vi "Remote Client.vi"(6 "Wait for Response? [T]":bool=TRUE, 8 "error in (no error)":errorcluster, 9 "Data":variant, 10 "Command":string, 11 "Instrument in":refnum<class "Instrument.lvclass">) -> (0 "error out":errorcluster, 1 "Data out":variant, 2 "Command out":string, 3 "Instrument out":refnum<class "Instrument.lvclass">)   [LabVIEW 2016, in "Instrument.lvclass"]
uses:
  Instrument.lvclass
  Instrument.lvclass/Instrument.ctl
  RemoteControl/RemoteControl.lvclass
  RemoteControl.STM/RemoteControl.STM.lvclass
  C:/user/patrick/hg/levylab_inst/lvsrc/SMOs/RemoteControl/RemoteControl.lvclass
  <userlib>/_OpenG.lib/numeric/numeric.llb/Random Number Within Range - I32__ogtk.vi
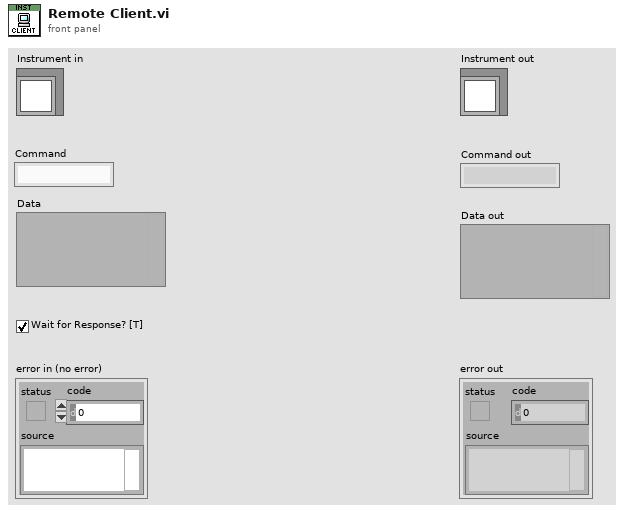
[diagram p1: front panel]
types:
  T1 = typedef "Instrument.lvclass/PublicEvents--Cluster.ctl" = cluster{"MessageFromProcess":refnum<user-event>}
  T2 = typedef "Instrument.lvclass/SMO RC Type--enum.ctl" = enum16{"RC", "STM", "ZMQ"}
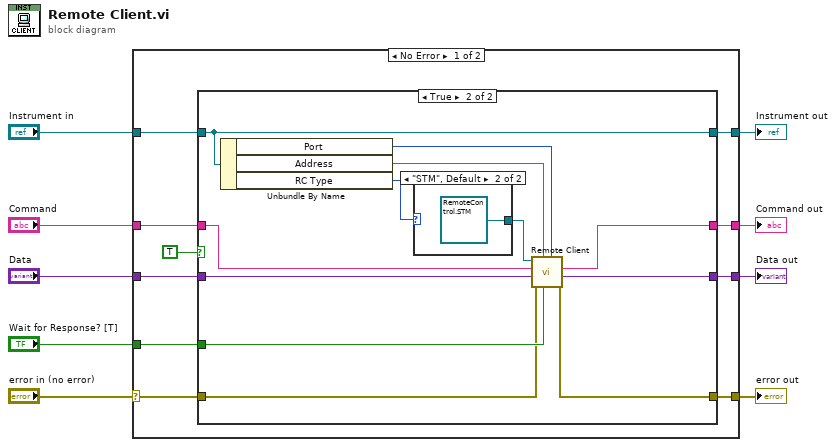
[diagram p0: block diagram]
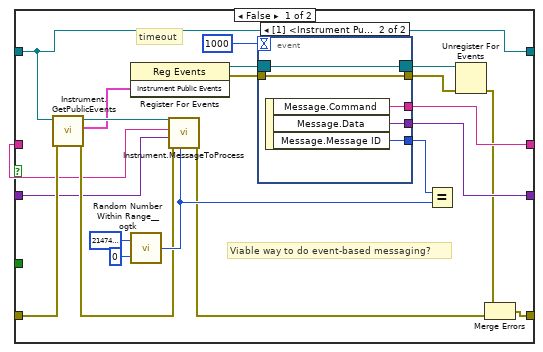
[diagram p2: hidden frame]
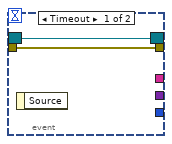
[diagram p3: hidden frame]
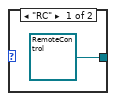
[diagram p4: hidden frame]
diagram:
  n1 = case shown="No Error" "error in (no error)" {
    selector: "error in (no error)" -> [w19 w64]
    tunnel: [w18 w64] -> w8
    tunnel: [w10 w63] -> w6
    tunnel: "Instrument in" -> [w11 w63]
    tunnel: [w17 _] -> w5
    tunnel: [w13 w62] -> w4
    tunnel: "Command" -> [w14 w62]
    tunnel: "Data" -> [w16 _]
    tunnel: "Wait for Response? [T]" -> [w15 _]
    frame No Error {
      n2 = case shown="True" TRUE {
        tunnel: w19 -> [w29 w52]
        tunnel: [w22 w59] -> w18
        tunnel: [w35 w58] -> w17
        tunnel: w16 -> [w27 w57]
        tunnel: w15 -> [_ w56]
        tunnel: w11 -> [w20 w48]
        tunnel: w14 -> [w26 w53]
        tunnel: [w25 w54] -> w13
        tunnel: [w20 w48] -> w10
        frame False {
          # "Viable way to do event-based messaging?"
          # "timeout"
          n3 = call "Instrument.GetPublicEvents.vi"("error in (no error)"=w29, "Instrument"=w20) -> ("error out"=w28:errorcluster, "Instrument Public Events"=w37:T1, "Instrument out"=w38:refnum<class "Instrument.lvclass">)  [unwired: 7 in]
          n4 = register-events(w37) -> (reference out=w36:refnum<event-registration>, error out=w32:errorcluster)  [unwired: 2 in]
          n5 = call-poly <userlib>:"Random Number Within Range__ogtk.vi"("High"=2147483647, "Low"=0) -> ("Random Number"=w31:i32)  [unwired: 3 in]
          n6 = call "Instrument.MessageToProcess.vi"("Message ID"=w31, "error in (no error)"=w28, "Message.Data"=w27, "Message.Command"=w26, "Instrument"=w38) -> ("error out"=w21:errorcluster)  [unwired: 5 in, 1 out]
          n7 = event shown="[1] <Instrument Public Events.MessageFromProcess>: User Event" {
            selector: w36 -> [w41 w43]
            dyn-events: [w41 w43] -> w24
            timeout: 1000 -> [_ _]
            tunnel: [_ w47] -> w25
            tunnel: [_ w46] -> w35
            tunnel: [w42 w45] -> w33
            tunnel: w32 -> [w42 w45]
            tunnel: [_ w44] -> w30
            event Timeout {
              n8 = event-data() -> ()  [unwired: 1 in, 1 out]
            }
            event User Event {
              n9 = event-data() -> ("Message.Command"=w47:string, "Message.Data"=w46:variant, "Message.Message ID"=w44:i32)  [unwired: 1 in]
            }
          }
          n10 = Equal?(x=w30, y=w31) -> ()  [unwired: 1 out]
          n11 = Unregister For Events(event registration refnum=w24, error in=w33) -> (error out=w23:errorcluster)
          n12 = Merge Errors(w23, w21) -> (w22:errorcluster)
        }
        frame True {
          n13 = Unbundle By Name(w48) -> ("Port"=w51:u16, "Address"=w55:string, "RC Type"=w49:T2)
          n14 = case shown="\"STM\", Default" w49 {
            tunnel: [refnum<class "RemoteControl.lvclass"> refnum ("RemoteControl in") refnum<class "RemoteControl.STM.lvclass"> refnum ("RemoteControl.STM.lvclass")] -> w50
            frame "RC" {
            }
            frame "STM", Default {
            }
          }
          n15 = call "Remote Client.vi"("Port"=w51, "Wait for Response?"=w56, "address"=w55, "error in (no error)"=w52, "Data"=w57, "Command"=w53, "RemoteControl in"=w50) -> ("error out"=w59:errorcluster, "Data out"=w58:variant, "Command out"=w54:string)  [unwired: 1 in, 1 out]
        }
      }
    }
    frame Error {
    }
  }
  "error out" <- w8
  "Instrument out" <- w6
  "Command out" <- w4
  "Data out" <- w5
